vi "Flatten Array Of Strings.vi"(7 "# Elements":i32, 10 "Array of Strings":string[](array[string])) -> (2 "Flattened String":string)   [LabVIEW 2024]
panel:
  # "Flattens an array of strings by concatonating in order with a\ncomma between each original string element."
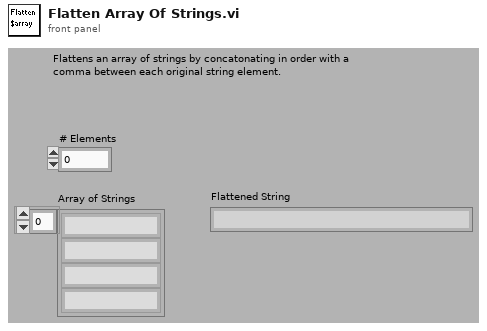
[diagram p1: front panel]
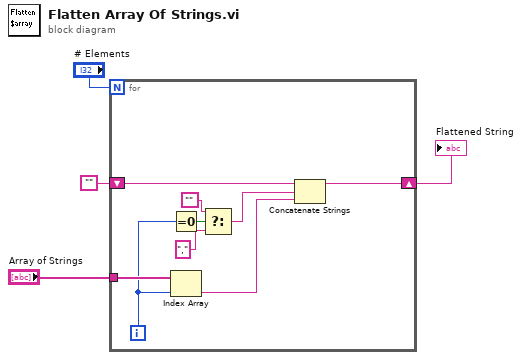
[diagram p0: block diagram]
diagram:
  n1 = for {
    N: "# Elements" -> [_]
    shift-right: [w5] -> w1
    shift-left: "" -> [w10]
    tunnel: "Array of Strings" -> [w13]
    i -> [w9]
    n2 = Equal To 0?(x=w9) -> (x = 0?=w12:bool)
    n3 = Index Array(array=w13, index=w9) -> (element=w6:string)
    n4 = Select(t="", s=w12, f=",") -> (s? t:f=w7:string)
    n5 = Concatenate Strings(w10, w7, w6) -> (w5:string)
  }
  "Flattened String" <- w1
